vi "Tabor 5064 Control.vi"() -> ()   [LabVIEW 2018]
panel:
  in  "set_phases":bool
  out "ramping":bool
  out "rate (Hz / s)":dbl
  in  "step_size (Hz)":dbl format="%#_13g"
  in  "final_frequency (Hz)":dbl format="%#_13g"
  in  "ramp_frequency":bool
  in  "loop timer (ms)":u32=500
  out "freqs":dbl[](array[numeric])
  in  "set_frequency":bool
  out "user_phases":dbl[](array[numeric])=[0.0, 180.0, 0.0, 0.0]
  out "user_offsets":dbl[](array[numeric])
  out "user_amps":dbl[](array[numeric])=[2.0, 2.0, 0.01, 0.01]
  in  "set_amplitudes":bool
  out "ch_status":bool[](array[boolean])=[TRUE, TRUE, FALSE, FALSE]
  in  "get_channel_state":bool
  in  "ch4_load":u32=10000
  in  "ch3_load":u32=10000
  in  "ch2_load":u32=10000
  in  "ch1_load":u32=10000
  in  "set_channel_load":bool
  in  "ch4_on":bool
  in  "ch3_on":bool
  in  "ch2_on":bool=TRUE
  in  "ch1_on":bool=TRUE
  in  "set_channel_enable":bool
  out "offsets":dbl[](array[numeric])
  in  "independent_offset?":bool
  in  "ch4_offset":dbl format="%#_13g"
  in  "ch3_offset":dbl format="%#_13g"
  in  "ch2_offset":dbl format="%#_13g"
  in  "ch1_offset":dbl format="%#_13g"
  out "phases":dbl[](array[numeric])=[0.0, 180.0, 0.0, 0.0]
  in  "independent_phase?":bool=TRUE
  in  "ch4_phase":dbl format="%#_13g"
  in  "ch3_phase":dbl format="%#_13g"
  in  "ch2_phase":dbl=180.0 format="%#_13g"
  in  "ch1_phase":dbl format="%#_13g"
  in  "GPIB Address":string="4"
  out "amps":dbl[](array[numeric])=[2.0, 2.0, 0.01, 0.01]
  in  "independent_amp?":bool=TRUE
  in  "waveform_freq (Hz)":dbl=41.0 format="%#_13g"
  in  "ch4_amp":dbl=0.01 format="%#_13g"
  in  "ch3_amp":dbl=0.01 format="%#_13g"
  in  "ch2_amp":dbl=2.0 format="%#_13g"
  in  "ch1_amp":dbl=2.0 format="%#_13g"
  in  "setup_channels":bool
  # "AMPLITUDES ARE PEAK-TO-PEAK"
  # "USUAL PHASE:\n0\n180\n270\n90"
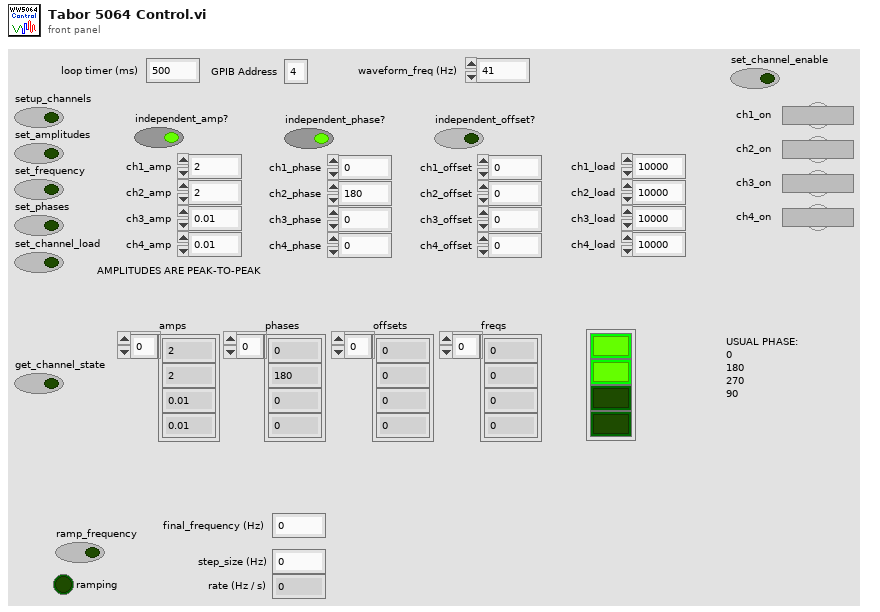
[diagram p1: front panel]
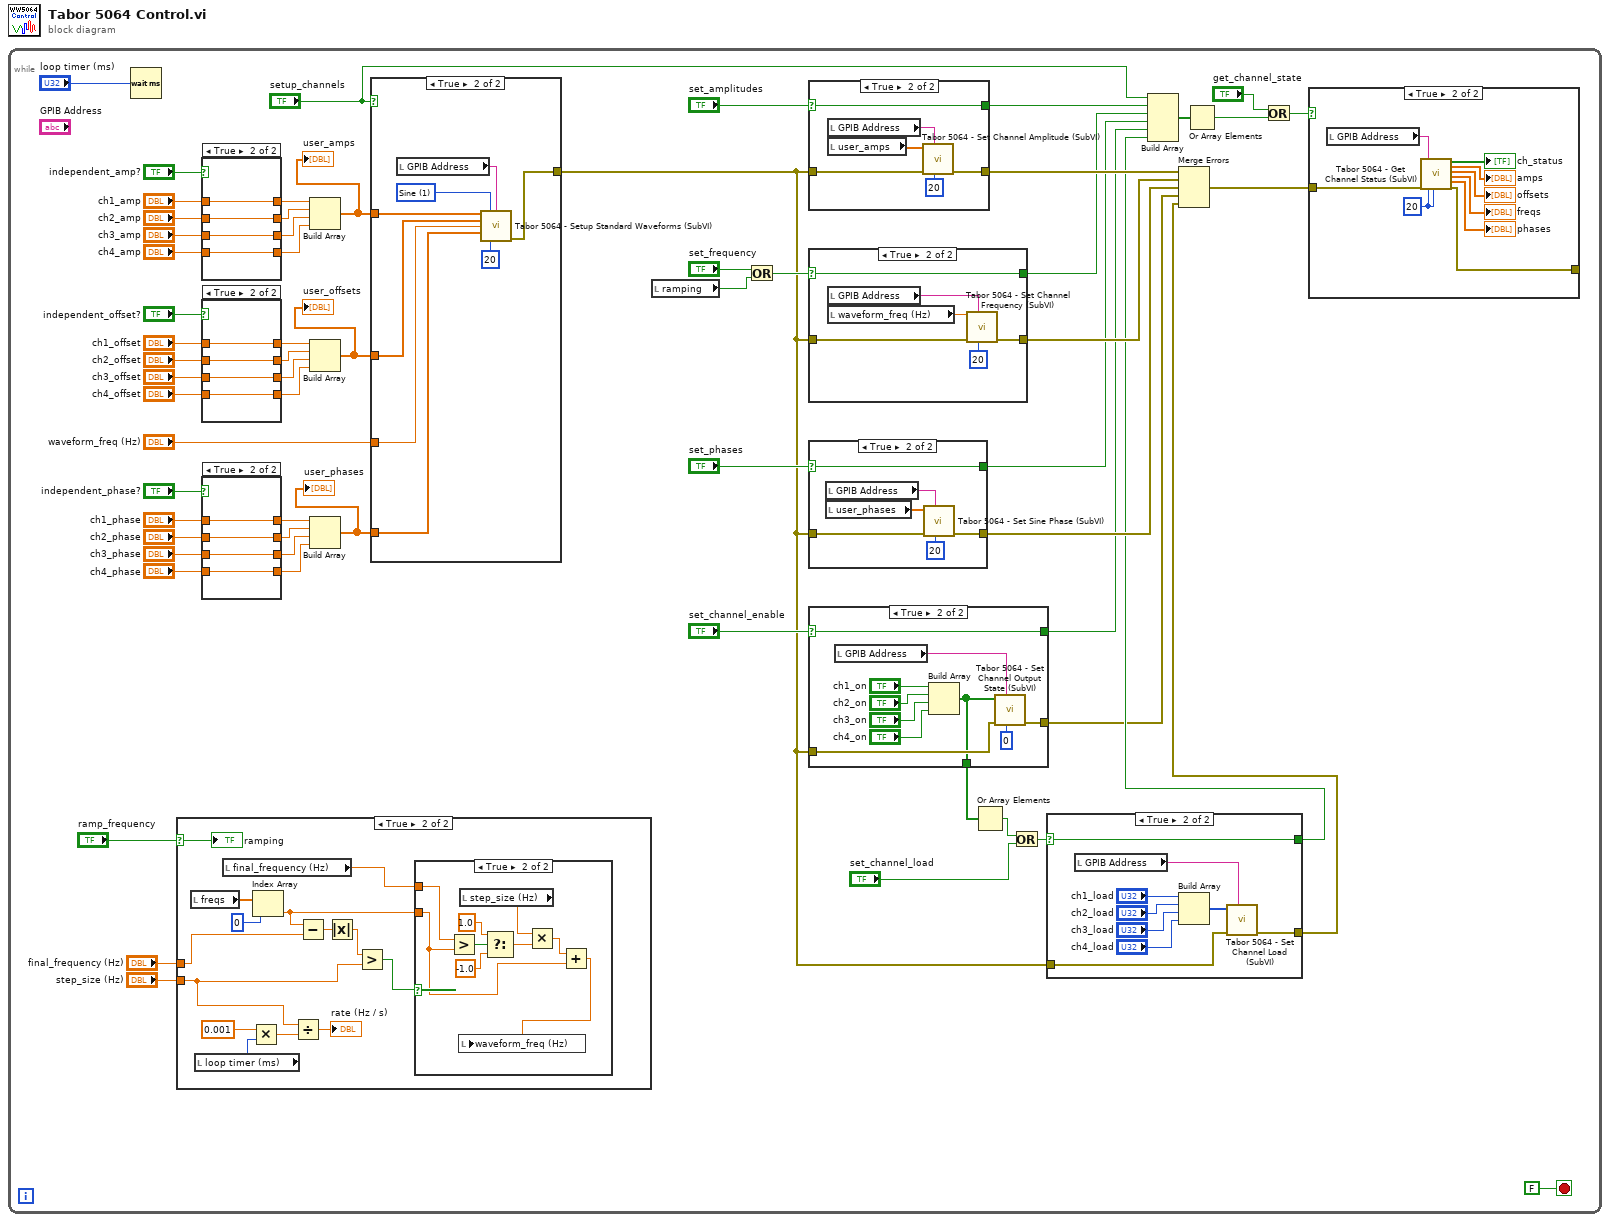
[diagram p0: block diagram]
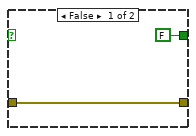
[diagram p2: hidden frame]
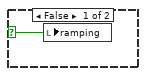
[diagram p3: hidden frame]
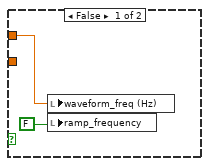
[diagram p4: hidden frame]
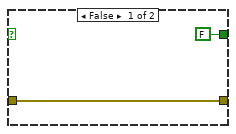
[diagram p5: hidden frame]
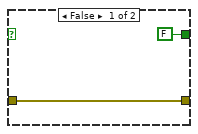
[diagram p6: hidden frame]
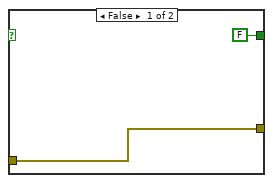
[diagram p8: hidden frame]
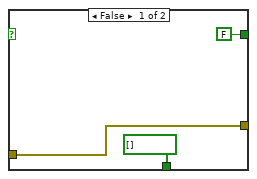
[diagram p9: hidden frame]
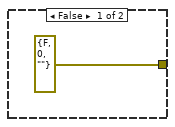
[diagram p13: hidden frame]
diagram:
  n1 = while {
    stop <- FALSE stop-if-true
    n2 = Wait (ms)(milliseconds to wait="loop timer (ms)") -> ()  [unwired: 1 out]
    n3 = case shown="True" "ramp_frequency" {
      selector: "ramp_frequency" -> [w72 w78]
      tunnel: "final_frequency (Hz)" -> [_ w80]
      tunnel: "step_size (Hz)" -> [_ w77]
      frame False {
        n4 = local write "ramping"(w72) -> ()
      }
      frame True {
        n5 = local read "freqs"() -> (w82:dbl[])
        n6 = local read "loop timer (ms)"() -> (w85:u32)
        n7 = local read "final_frequency (Hz)"() -> (w74:dbl)
        n8 = Multiply(x=0.001, y=w85) -> (x*y=w84:dbl)
        n9 = Index Array(array=w82, index=0) -> (element=w75:dbl)
        n10 = Divide(x=w77, y=w84) -> (x/y=→"rate (Hz / s)":dbl)
        n11 = Subtract(x=w75, y=w80) -> (x-y=w79:dbl)
        n12 = Absolute Value(x=w79) -> (abs(x)=w76:dbl)
        n13 = Greater?(x=w76, y=w77) -> (0:w73:bool)
        n14 = case shown="True" w73 {
          tunnel: w75 -> [_ w90]
          tunnel: w74 -> [w87 w97]
          frame False {
            n15 = local write "waveform_freq (Hz)"(w87) -> ()
            n16 = local write "ramp_frequency"(FALSE) -> ()
          }
          frame True {
            n17 = Greater?(x=w97, y=w90) -> (0:w96:bool)
            n18 = local read "step_size (Hz)"() -> (w93:dbl)
            n19 = Select(t=1.0, s=w96, f=-1.0) -> (s? t:f=w92:dbl)
            n20 = Multiply(x=w93, y=w92) -> (x*y=w91:dbl)
            n21 = Add(x=w91, y=w90) -> (x+y=w89:dbl)
            n22 = local write "waveform_freq (Hz)"(w89) -> ()
          }
        }
        "ramping" <- w78
      }
    }
    n23 = case shown="True" "independent_amp?" {
      tunnel: [w158 w162] -> w53
      tunnel: "ch1_amp" -> [w158 w162]
      tunnel: [w158 w161] -> w60
      tunnel: "ch2_amp" -> [_ w161]
      tunnel: [w158 w160] -> w59
      tunnel: "ch3_amp" -> [_ w160]
      tunnel: [w158 w159] -> w58
      tunnel: "ch4_amp" -> [_ w159]
      frame False {
      }
      frame True {
      }
    }
    n24 = case shown="True" "independent_offset?" {
      tunnel: [w148 w152] -> w34
      tunnel: "ch1_offset" -> [w148 w152]
      tunnel: [w148 w151] -> w41
      tunnel: "ch2_offset" -> [_ w151]
      tunnel: [w148 w150] -> w40
      tunnel: "ch3_offset" -> [_ w150]
      tunnel: [w148 w149] -> w39
      tunnel: "ch4_offset" -> [_ w149]
      frame False {
      }
      frame True {
      }
    }
    n25 = case shown="True" "independent_phase?" {
      tunnel: [w153 w157] -> w43
      tunnel: "ch1_phase" -> [w153 w157]
      tunnel: [w153 w156] -> w50
      tunnel: "ch2_phase" -> [_ w156]
      tunnel: [w153 w155] -> w49
      tunnel: "ch3_phase" -> [_ w155]
      tunnel: [w153 w154] -> w48
      tunnel: "ch4_phase" -> [_ w154]
      frame False {
      }
      frame True {
      }
    }
    n26 = Build Array(w53, w60, w59, w58) -> (w30:dbl[])
    "user_amps" <- w30
    n27 = Build Array(w34, w41, w40, w39) -> (w29:dbl[])
    "user_offsets" <- w29
    n28 = Build Array(w43, w50, w49, w48) -> (w28:dbl[])
    "user_phases" <- w28
    n29 = case shown="True" "setup_channels" {
      tunnel: w30 -> [_ w170]
      tunnel: "waveform_freq (Hz)" -> [_ w168]
      tunnel: w28 -> [_ w167]
      tunnel: w29 -> [_ w169]
      tunnel: [errorcluster {"status"=FALSE, "code"=0, "source"=""} ("error_out") w164] -> w9
      frame False {
      }
      frame True {
        w165 = u16 1 items=["DC", "Sine", "Triangle", "Square"] ("waveform_type")
        n30 = local read "GPIB Address"() -> (w171:string)
        n31 = call "Tabor 5064 - Setup Standard Waveforms (SubVI).vi"("amps (V)"=w170, "waveform_type"=w165, "GPIB Address"=w171, "offsets (V)"=w169, "freq"=w168, "phases (deg)"=w167, "write_delay (ms)"=u32 20) -> ("error_out"=w164:errorcluster)  [unwired: 8 in]
      }
    }
    n32 = local read "ramping"() -> (w13:bool)
    n33 = Or(x="set_frequency", y=w13) -> (x .or. y?=w17:bool)
    n34 = case shown="True" "set_amplitudes" {
      selector: "set_amplitudes" -> [_ w108]
      tunnel: w9 -> [w107 w112]
      tunnel: [w107 w111] -> w27
      tunnel: [FALSE w108] -> w23
      frame False {
      }
      frame True {
        n35 = local read "GPIB Address"() -> (w113:string)
        n36 = local read "user_amps"() -> (w110:dbl[])
        n37 = call "Tabor 5064 - Set Channel Amplitude (SubVI).vi"("write_delay (ms)"=u32 20, "GPIB Address"=w113, "error_in"=w112, "amps (V)"=w110) -> ("error_out"=w111:errorcluster)  [unwired: 7 in]
      }
    }
    n38 = case shown="True" w17 {
      selector: w17 -> [_ w100]
      tunnel: w9 -> [w99 w101]
      tunnel: [w99 w103] -> w25
      tunnel: [FALSE w100] -> w22
      frame False {
      }
      frame True {
        n39 = local read "GPIB Address"() -> (w105:string)
        n40 = local read "waveform_freq (Hz)"() -> (w102:dbl)
        n41 = call "Tabor 5064 - Set Channel Frequency (SubVI).vi"("write_delay (ms)"=u32 20, "GPIB Address"=w105, "error_in"=w101, "frequency"=w102) -> ("error_out"=w103:errorcluster)  [unwired: 7 in]
      }
    }
    n42 = case shown="True" "set_phases" {
      selector: "set_phases" -> [_ w71]
      tunnel: [FALSE w71] -> w11
      tunnel: w9 -> [w64 w67]
      tunnel: [w64 w66] -> w10
      frame False {
      }
      frame True {
        n43 = local read "GPIB Address"() -> (w69:string)
        n44 = local read "user_phases"() -> (w70:dbl[])
        n45 = call "Tabor 5064 - Set Sine Phase (SubVI).vi"("write_delay (ms)"=u32 20, "GPIB Address"=w69, "error_in"=w67, "phases (deg)"=w70) -> ("error_out"=w66:errorcluster)  [unwired: 7 in]
      }
    }
    n46 = case shown="True" "set_channel_enable" {
      selector: "set_channel_enable" -> [_ w140]
      tunnel: w9 -> [w137 w142]
      tunnel: [w137 w141] -> w2
      tunnel: [FALSE w140] -> w8
      tunnel: [bool[] [] w139] -> w4
      frame False {
      }
      frame True {
        n47 = local read "GPIB Address"() -> (w143:string)
        n48 = Build Array("ch1_on", "ch2_on", "ch3_on", "ch4_on") -> (w139:bool[])
        n49 = call "Tabor 5064 - Set Channel Output State (SubVI).vi"("write_delay (ms)"=u32 0, "GPIB Address"=w143, "error_in"=w142, "ch_enable"=w139) -> ("error_out"=w141:errorcluster)  [unwired: 7 in]
      }
    }
    n50 = Or Array Elements(Boolean array=w4) -> (logical OR=w5:bool)
    n51 = Or(x=w5, y="set_channel_load") -> (x .or. y?=w6:bool)
    n52 = case shown="True" w6 {
      selector: w6 -> [_ w126]
      tunnel: w9 -> [w125 w128]
      tunnel: [w125 w127] -> w1
      tunnel: [FALSE w126] -> w7
      frame False {
      }
      frame True {
        n53 = local read "GPIB Address"() -> (w129:string)
        n54 = Build Array("ch1_load", "ch2_load", "ch3_load", "ch4_load") -> (w130:u32[])
        n55 = call "Tabor 5064 - Set Channel Load (SubVI).vi"("GPIB Address"=w129, "error_in"=w128, "channel_loads"=w130) -> ("error_out"=w127:errorcluster)  [unwired: 8 in]
      }
    }
    n56 = Build Array("setup_channels", w23, w22, w11, w8, w7) -> (w21:bool[])
    n57 = Merge Errors(w27, w25, w10, w2, w1) -> (w26:errorcluster)
    n58 = Or Array Elements(Boolean array=w21) -> (logical OR=w20:bool)
    n59 = Or(x="get_channel_state", y=w20) -> (x .or. y?=w33:bool)
    n60 = case shown="True" w33 {
      tunnel: w26 -> [w114 w123]
      tunnel: [w114 w120] -> _
      frame False {
      }
      frame True {
        w115 = u32 20 ("write_delay (ms)")
        n61 = local read "GPIB Address"() -> (w122:string)
        n62 = call "Tabor 5064 - Get Channel Status (SubVI).vi"("error_in"=w123, "GPIB Address"=w122, "write_delay (ms)"=w115, "read_delay (ms)"=w115) -> ("ch_status"=→"ch_status":bool[], "amps"=→"amps":dbl[], "offsets"=→"offsets":dbl[], "freqs"=→"freqs":dbl[], "phases"=→"phases":dbl[], "error_out"=w120:errorcluster)  [unwired: 10 in]
      }
    }
  }
